vi "VIsReplaced.vi"() -> ()   [LabVIEW 2016, in "SwitchDependenciesVariables.lvlib"]
uses:
  SwitchDependenciesVariables.lvlib
panel:
  in  "VIsReplaced":string
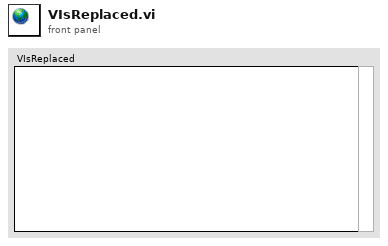
[diagram p1: front panel]
diagram:
